vi "CloseCom.vi"(11 "error in (no error)":errorcluster) -> (15 "error out":errorcluster)   [LabVIEW 2009]
uses:
  globals/VISAResourceName.vi
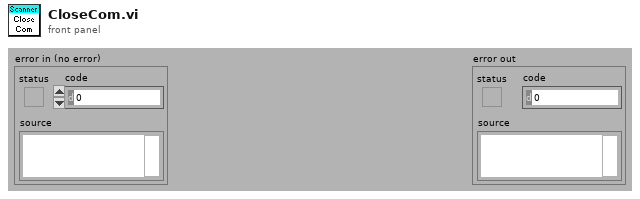
[diagram p1: front panel]
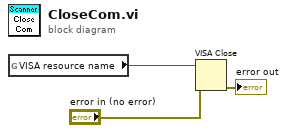
[diagram p0: block diagram]
diagram:
  n1 = global read "VISAResourceName.vi" "VISA resource name"() -> (w3:refnum<visa-resource-name>)
  n2 = VISA Close(VISA resource name=w3, error in (no error)="error in (no error)") -> (error out=→"error out":errorcluster)
